vi "cook.vi"(8 "error in (no error)":errorcluster, 11 "Simmer in":refnum<class "Simmer.lvclass">) -> (0 "error out":errorcluster, 3 "Simmer out":refnum<class "Simmer.lvclass">)   [LabVIEW 2011, in "CookBehaviors.lvlib" / "Simmer.lvclass"]
uses:
  Simmer.lvclass
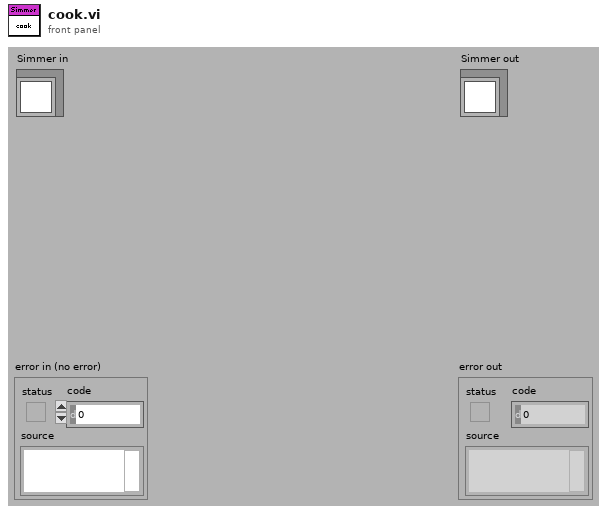
[diagram p1: front panel]
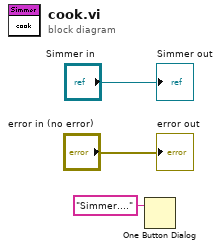
[diagram p0: block diagram]
diagram:
  n1 = One Button Dialog(message="Simmer....") -> ()  [unwired: 1 in, 1 out]
  "error out" <- "error in (no error)"
  "Simmer out" <- "Simmer in"
